vi "test_FXP Unsigned Value Conversion_0+delta.vi"(8 "error in (no error)":errorcluster, 11 "TestCase in":refnum<class "FPGA Register IO Tests.lvclass">) -> (0 "error out":errorcluster, 3 "TestCase out":refnum<class "FPGA Register IO Tests.lvclass">)   [LabVIEW 2021, in "FPGA Register IO Tests.lvclass"]
uses:
  FPGA Register IO Tests.lvclass
  APIs/FPGA Register IO/TypeDefs/FXP Configuration.ctl
  <vilib>/fxp/LVFixedPointRepBitsTypeDef.ctl
  <vilib>/fxp/LVFixedPointRepRangeTypeDef.ctl
  <vilib>/addons/_JKI Toolkits/VI Tester/TestCase.llb/TestCase.lvclass
  APIs/FPGA Register IO/FPGA Register IO.lvlib
  <vilib>/Utility/Data Type/NI_Data Type.lvlib
  C:/Program Files/National Instruments/LabVIEW 2021/vi.lib/addons/_JKI Toolkits/VI Tester/TestCase.llb/TestCase.lvclass
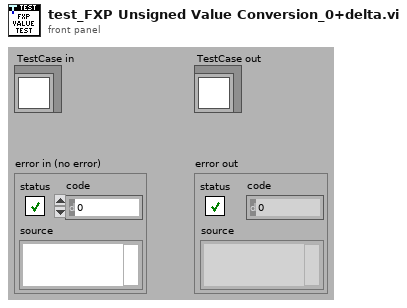
[diagram p1: front panel]
types:
  T1 = typedef "FPGA Register IO.lvlib/FXP Configuration.ctl" = cluster{"FXP Representation":T2, "FXP Range":T3}
  T2 = typedef "LVFixedPointRepBitsTypeDef.ctl" = cluster{"Signed":bool, "Word Length":u32, "Integer Word Length":i32}
  T3 = typedef "LVFixedPointRepRangeTypeDef.ctl" = cluster{"Range Min":dbl, "Range Max":dbl, "Delta":dbl}
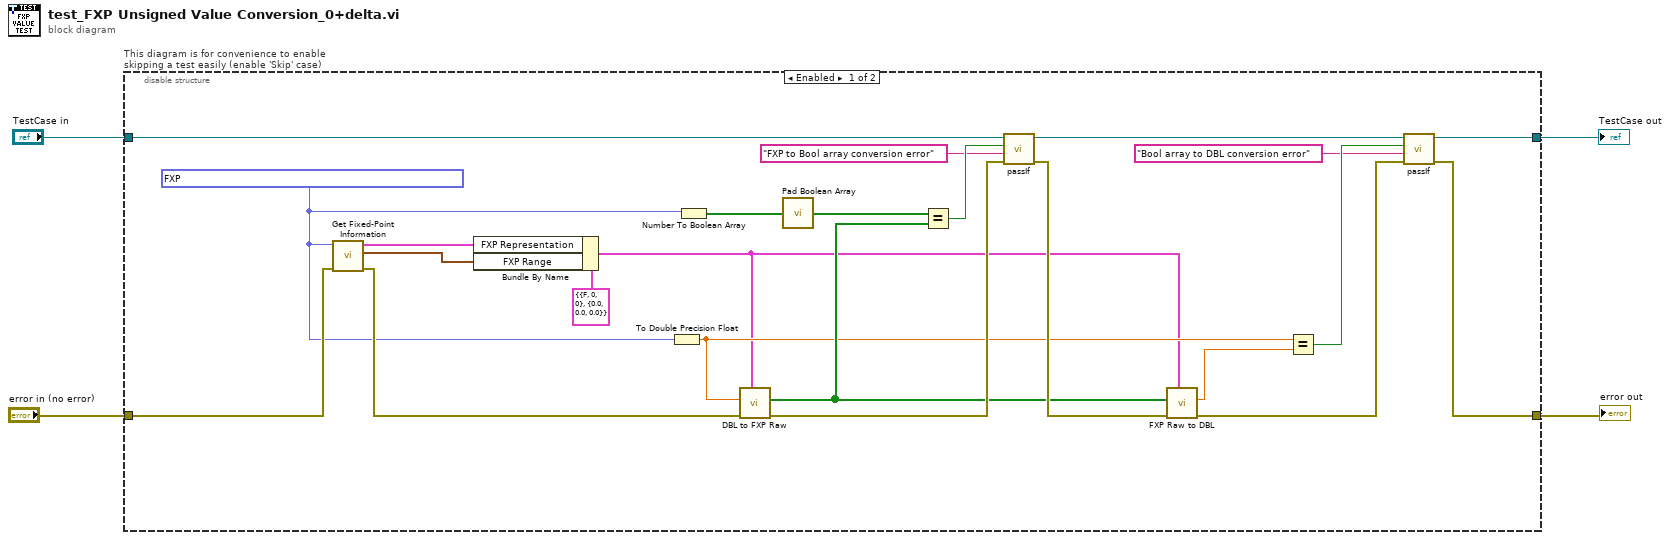
[diagram p0: block diagram]
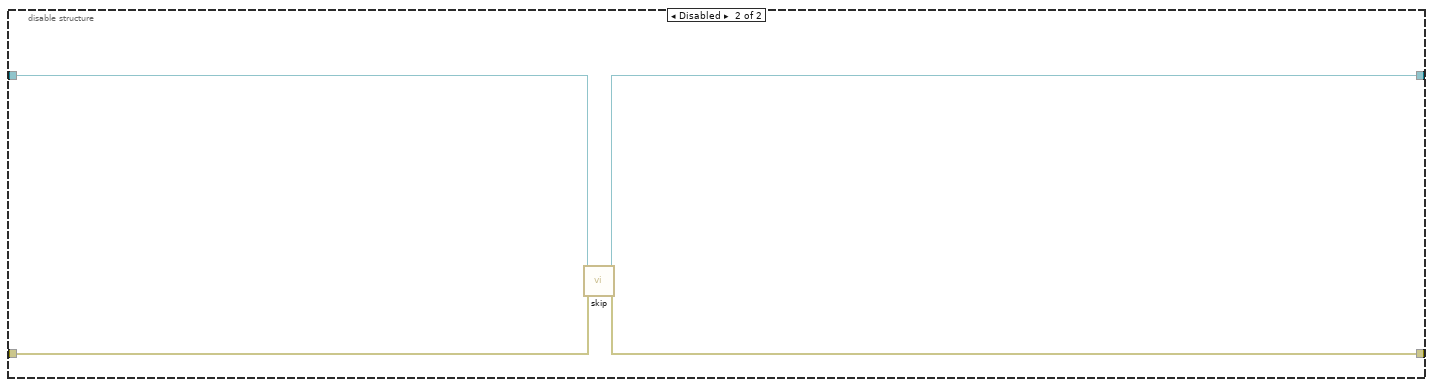
[diagram p2: hidden frame]
diagram:
  n1 = disable-structure "This diagram is for convenience to enable skipping a test easily (enable 'Skip' case)" shown="Enabled" {
    disable-tunnel: "TestCase in" -> [w27 w31]
    disable-tunnel: [w17 w29] -> w1
    disable-tunnel: [w18 w30] -> w3
    disable-tunnel: "error in (no error)" -> [w9 w28]
    frame Enabled {
      w7 = fxp<+,64,1> 1.0842021724855044e-19
      n2 = call <vilib>:"Get Fixed-Point Information.vi"("error in (no error)"=w9, "variant"=w7) -> ("error out"=w8:errorcluster, "FXP range"=w10:T3, "FXP representation"=w11:T2)  [unwired: 6 in, 1 out]
      n3 = Bundle By Name(cluster=T1 {"FXP Representation"={"Signed"=FALSE, "Word Length"=0, "Integer Word Length"=0}, "FXP Range"={"Range Min"=0.0, "Range Max"=0.0, "Delta"=0.0}} ("FXP Configuration"), "FXP Representation"=w11, "FXP Range"=w10) -> (w12:T1)
      n4 = To Double Precision Float(number=w7) -> (double precision float=w14:dbl)
      n5 = Number To Boolean Array(number=w7) -> (Boolean array=w6:bool[])
      n6 = call "DBL to FXP Raw.vi"("FXP Configuration"=w12, "error in (no error)"=w8, "DBL Value"=w14) -> ("error out"=w26:errorcluster, "Bool Data"=w22:bool[])  [unwired: 7 in]
      n7 = call "Pad Boolean Array.vi"("Boolean array in"=w6) -> ("Padded array"=w5:bool[])
      n8 = Equal?(x=w5, y=w22) -> (x = y?=w25:bool)
      n9 = call-dynamic "passIf.vi"("error in (no error)"=w26, "message (\"\")"="FXP to Bool array conversion error" ("message (\"\")"), "pass"=w25, "TestCase in"=w27) -> ("error out"=w24:errorcluster, "TestCase out"=w21:refnum<class "FPGA Register IO Tests.lvclass">)  [unwired: 6 in]
      n10 = call "FXP Raw to DBL.vi"("FXP Configuration"=w12, "error in (no error)"=w24, "Bool Data"=w22) -> ("error out"=w19:errorcluster, "DBL Value"=w15:dbl)  [unwired: 7 in]
      n11 = Equal?(x=w14, y=w15) -> (x = y?=w20:bool)
      n12 = call-dynamic "passIf.vi"("error in (no error)"=w19, "message (\"\")"="Bool array to DBL conversion error" ("message (\"\")"), "pass"=w20, "TestCase in"=w21) -> ("error out"=w18:errorcluster, "TestCase out"=w17:refnum<class "FPGA Register IO Tests.lvclass">)  [unwired: 6 in]
    }
    frame Disabled {
      # "skip test result while test is under development"
      n13 = call <vilib>:"skip.vi"("error in (no error)"=w28, "TestCase in"=w31) -> ("error out"=w30:errorcluster, "TestCase out"=w29:refnum<class "FPGA Register IO Tests.lvclass">)  [unwired: 8 in]
    }
  }
  "error out" <- w3
  "TestCase out" <- w1
